vi "Configure AnalogOut Channel.vi"(0 "ADALM2000 Handler":u64 caption="Instrument Handle Out", 5 "Channel":T1, 7 "Samplerate":T2, 9 "Enable":bool, 11 "Cyclic":bool) -> (4 "ADALM2000 Handler 2":u64 caption="Instrument Handle Out")   [LabVIEW 2022 SP3]
uses:
  Controls/SampleRateControlOut.ctl
  Controls/AnalogChannel.ctl
  libm2k_lv.dll
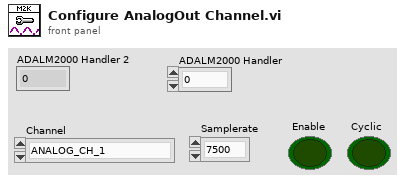
[diagram p1: front panel]
types:
  T1 = typedef "AnalogChannel.ctl" = enum16{"ANALOG_CH_1", "ANALOG_CH_2"}
  T2 = typedef "SampleRateControlOut.ctl" = enum16{"7500", "75000", "750000", "7500000", "75000000"}
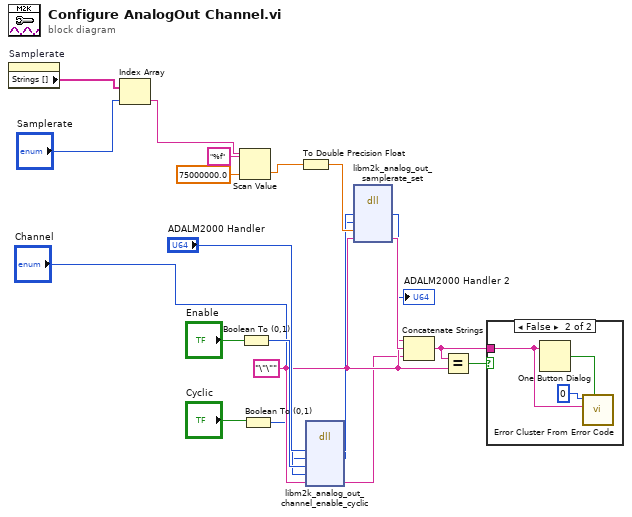
[diagram p0: block diagram]
diagram:
  w11 = "\"\""
  n1 = property on="Samplerate" class="Enum (strict)"() -> ("Strings []"=w6:string[])  [unwired: 2 in, 2 out]
  n2 = Index Array(array=w6, index="Samplerate") -> (element=w1:string)
  n3 = Scan Value(string=w1, format string="%f", default (0 dbl)=75000000.0) -> (value=w2:dbl)  [unwired: 1 out]
  n4 = Boolean To (0,1)(Boolean="Enable") -> (0, 1=w13:i16)
  n5 = Boolean To (0,1)(Boolean="Cyclic") -> (0, 1=w8:i16)
  n6 = To Double Precision Float(number=w2) -> (double precision float=w21:dbl)
  n7 = dll-call lib="libm2k_lv.*" fn="libm2k_analog_out_channel_enable_cyclic"("instance"="ADALM2000 Handler", "chnIdx"="Channel", "enable"=w13, "cyclic"=w8, "err"=w11) -> ("instance"=w16:u64, "chnIdx"=w14:u64, "err"=w10:string)  [unwired: 6 in, 2 out]
  n8 = dll-call lib="libm2k_lv.*" fn="libm2k_analog_out_samplerate_set"("instance"=w16, "chnIdx"=w14, "samplerate"=w21, "err"=w11) -> ("instance"=→"ADALM2000 Handler 2":u64, "err"=w20:string)  [unwired: 6 in, 2 out]
  n9 = Concatenate Strings(w11, w20, w10) -> (w18:string)
  n10 = Equal?(x=w18, y=w11) -> (x = y?=w19:bool)
  n11 = case shown="False" w19 {
    tunnel: w18 -> [_ w22]
    frame True {
    }
    frame False {
      n12 = One Button Dialog(message=w22) -> (true=w24:bool)  [unwired: 1 in]
      n13 = call <vilib>:"Error Cluster From Error Code.vi"("show call chain? (False)"=w24, "error message (\"\")"=w22, "error code (0)"=0) -> ()  [unwired: 6 in, 1 out]
    }
  }
